vi "Test Customer with Phone Make Call Broadcasts Status.vi"(8 "error in (no error)":errorcluster, 11 "Customer With Phone Test In":refnum<class "Customer With Phone Test.lvclass">) -> (0 "error out":errorcluster, 3 "Customer With Phone Test Out":refnum<class "Customer With Phone Test.lvclass">)   [LabVIEW 2020, in "Customer With Phone Test.lvclass"]
uses:
  Customer With Phone Test.lvclass
  C:/Program Files (x86)/National Instruments/LabVIEW 2020/vi.lib/Astemes/LUnit/Test Case.lvclass
  Processes/People/Customers/Customer With Phone/Customer With Phone.lvclass
  C:/Program Files (x86)/National Instruments/LabVIEW 2020/vi.lib/Astemes/Triarc Framework/Process/Process.lvclass
  <vilib>/Astemes/Triarc Framework/Process/Process.lvclass/Process.ctl
  <vilib>/Astemes/LUnit/Test Case.lvclass/Test Case.ctl
  84041711-a98c-4458-8a7e-b29b434b9d89.vi
  <vilib>/Astemes/Triarc Framework/Process/Public/Lifecycle/Get Lifecycle State.vi
  <vilib>/Astemes/Triarc Framework/Support/Execution timer.vi
  <vilib>/Astemes/Triarc Framework/Process/Private/SubVIs/Wait for finish.vi
  <vilib>/Astemes/Triarc Framework/Process/Private/SubVIs/Set Lifecycle State.vi
  <vilib>/Astemes/Triarc Framework/Process/Protected/Messaging/Send Message.vi
  <vilib>/Astemes/LUnit/Append Pass Result.vi
  <vilib>/Astemes/LUnit/Append Fail Result.vi
  <vilib>/Astemes/LUnit/Describe Comparison.vi
  <vilib>/Astemes/LUnit/Compare Variants.vi
  <vilib>/Utility/error.llb/Clear Errors.vi
  <vilib>/Astemes/Triarc Framework/Process/Private/SubVIs/Handle Debug Data.vi
  <vilib>/Astemes/LUnit/Variant to string.vi
  <vilib>/Astemes/Triarc Framework/Logging/Log Debug.vi
  <vilib>/AdvancedString/1D String Array to Delimited String.vi
  <vilib>/Utility/High Resolution Relative Seconds.vi
  <vilib>/Utility/error.llb/Error Cluster From Error Code.vi
  <vilib>/Astemes/Triarc Framework/Support/Dequeue Broadcast Message.vi
  <vilib>/Astemes/Triarc Framework/Process/Public/Read Name.vi
  <vilib>/Utility/Data Type/Get Type Information.vi
  <vilib>/Utility/LVClass/Get LV Class Name.vi
  <vilib>/Astemes/Triarc Framework/Callback/Callback.lvclass
  <vilib>/Astemes/Triarc Framework/Process/Process.lvclass
  <vilib>/Astemes/Triarc Framework/Support/Broadcast Event Dequeuers.lvlib
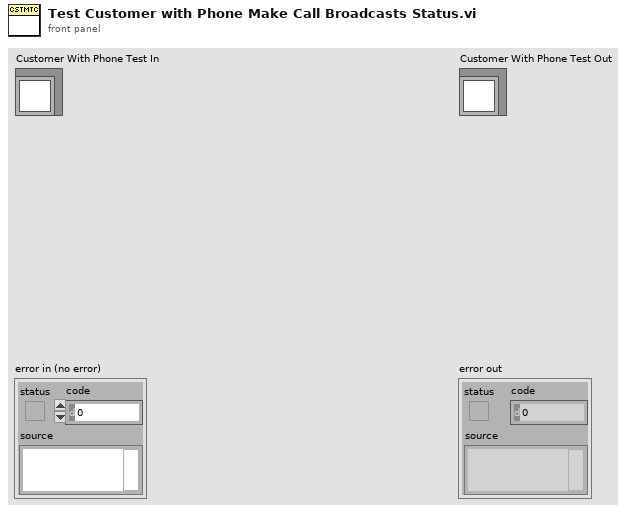
[diagram p1: front panel]
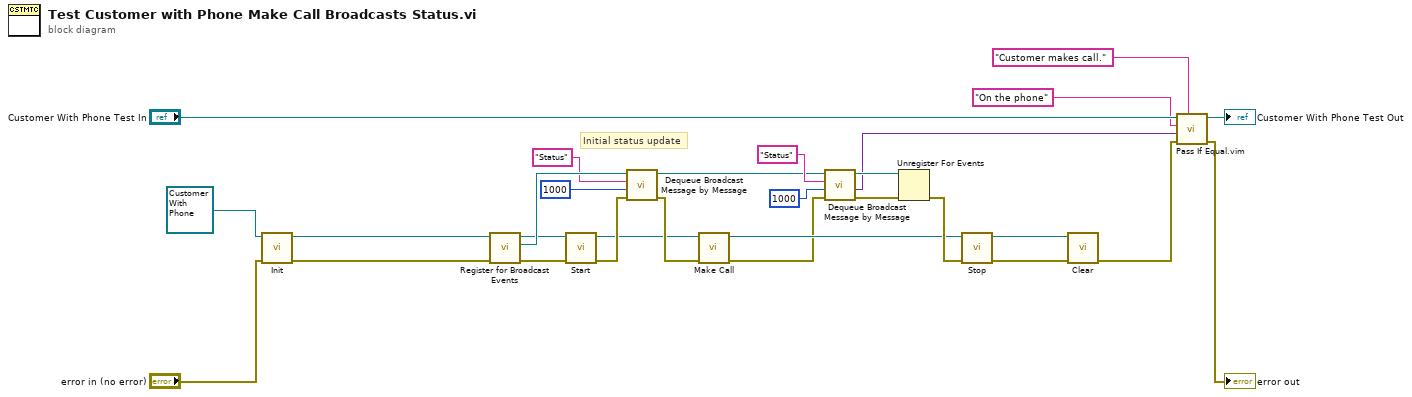
[diagram p0: block diagram]
diagram:
  # "Initial status update"
  n1 = call-dynamic "Init.vi"("error in (no error)"="error in (no error)", "View In"=refnum<class "Customer With Phone.lvclass"> refnum ("Customer With Phone.lvclass")) -> ("error out"=w29:errorcluster, "View Out"=w24:refnum<class "Customer With Phone.lvclass">)  [unwired: 8 in]
  n2 = call <vilib>:"Register for Broadcast Events.vi"("error in (no error)"=w29, "Process In"=w24) -> ("error out"=w6:errorcluster, "Event Registration Refnum Out"=w9:refnum<event-registration>, "Process Out"=w3:refnum<class "Customer With Phone.lvclass">)  [unwired: 7 in]
  n3 = call <vilib>:"Start.vi"("error in (no error)"=w6, "Process In"=w3) -> ("error out"=w4:errorcluster, "Process Out"=w2:refnum<class "Customer With Phone.lvclass">)  [unwired: 7 in, 1 out]
  n4 = call <vilib>:"Dequeue Broadcast Message by Message.vi"("error in (no error)"=w4, "Timeout (-1)"=1000, "Message"="Status", "Event Registration Refnum"=w9) -> ("error out"=w5:errorcluster, "Event Registration Refnum Out"=w8:refnum<event-registration>)  [unwired: 3 in, 3 out]
  n5 = call "Make Call.vi"("error in (no error)"=w5, "Customer With Phone In"=w2) -> ("error out"=w11:errorcluster, "Customer With Phone Out"=w27:refnum<class "Customer With Phone.lvclass">)  [unwired: 8 in]
  n6 = call <vilib>:"Dequeue Broadcast Message by Message.vi"("error in (no error)"=w11, "Timeout (-1)"=1000, "Message"="Status", "Event Registration Refnum"=w8) -> ("error out"=w10:errorcluster, "Message Data"=w14:variant, "Event Registration Refnum Out"=w15:refnum<event-registration>)  [unwired: 3 in, 2 out]
  n7 = Unregister For Events(event registration refnum=w15, error in=w10) -> (error out=w28:errorcluster)
  n8 = call <vilib>:"Stop.vi"("error in (no error)"=w28, "Process In"=w27) -> ("error out"=w26:errorcluster, "Process Out"=w25:refnum<class "Customer With Phone.lvclass">)  [unwired: 7 in, 1 out]
  n9 = call-dynamic "Clear.vi"("error in (no error)"=w26, "View In"=w25) -> ("error out"=w17:errorcluster)  [unwired: 9 in]
  n10 = call "Pass If Equal.vim"("Description"="Customer makes call.", "error in (no error)"=w17, "Actual"=w14, "Expected"="On the phone", "LUnit Test Case In"="Customer With Phone Test In") -> ("error out"=→"error out":errorcluster, "LUnit Test Case Out"=→"Customer With Phone Test Out":refnum<class "Customer With Phone Test.lvclass">)  [unwired: 5 in]
